vi "Parameterize Attributes.vi"(11 "Platform Application Attributes":T2[](array[typedef])) -> (2 "values":T1[](array[typedef]), 3 "attributes":T1[](array[typedef]))   [LabVIEW 2015, in "NI_AWS_SNS.lvlib" / "Platform Application.lvclass"]
uses:
  Platform Application.lvclass
  Application Attribute Value Pair.ctl
  Application Attribute.ctl
  Core/HTTP Request/Name Value Pair.ctl
  Core/HTTP Request/HTTP Request.lvclass
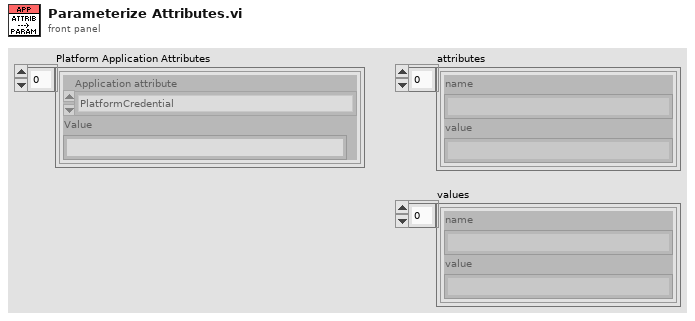
[diagram p1: front panel]
types:
  T1 = typedef "NI_AWS_Core.lvlib/HTTP Request.lvclass/Name Value Pair.ctl" = cluster{"name":string, "value":string}
  T2 = typedef "NI_AWS_SNS.lvlib/Platform Application.lvclass/Application Attribute Value Pair.ctl" = cluster{"Application attribute":T3, "Value":string}
  T3 = typedef "NI_AWS_SNS.lvlib/Platform Application.lvclass/Application Attribute.ctl" = enum16{"PlatformCredential", "PlatformPrincipal", "EventEndpointCreated", "EventEndpointDeleted", "EventEndpointUpdated", "EventDeliveryFailure", "SuccessFeedbackRoleArn", "FailureFeedbackRoleArn", "SuccessFeedbackSampleRate"}
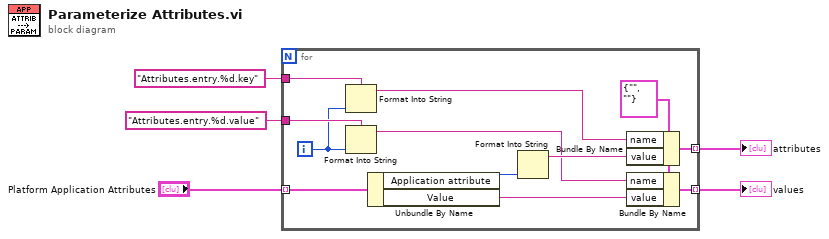
[diagram p0: block diagram]
diagram:
  n1 = for {
    tunnel: "Attributes.entry.%d.key" -> [w14]
    tunnel: "Attributes.entry.%d.value" -> [w12]
    tunnel: [w9] -> w3 mode=indexing
    tunnel: [w8] -> w4 mode=indexing
    tunnel: "Platform Application Attributes" -> [w6] mode=indexing
    i -> [w11]
    w7 = T1 {"name"="", "value"=""} ("element")
    n2 = Format Into String(format string=w14, w11) -> (resulting string=w13:string)  [unwired: 2 in, 1 out]
    n3 = Format Into String(format string=w12, w11) -> (resulting string=w10:string)  [unwired: 2 in, 1 out]
    n4 = Unbundle By Name(w6) -> ("Application attribute"=w17:T3, "Value"=w15:string)
    n5 = Format Into String(w17) -> (resulting string=w16:string)  [unwired: 3 in, 1 out]
    n6 = Bundle By Name(cluster=w7, "name"=w13, "value"=w16) -> (w9:T1)
    n7 = Bundle By Name(cluster=w7, "name"=w10, "value"=w15) -> (w8:T1)
  }
  "values" <- w4
  "attributes" <- w3
